vi "(SubVI)Scope_Down Sampling.vi"(7 "Init":bool, 9 "Sampling Time for Init":dbl format="%#_13g", 10 "Iteration":i32, 11 "Data In":i32[][](array[numeric])) -> (1 "end":bool, 2 "Loop Delay (sec)":dbl, 3 "Data Out":i32[][](array[numeric]))   [LabVIEW 2020]
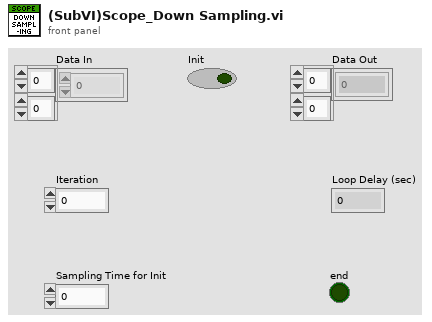
[diagram p1: front panel]
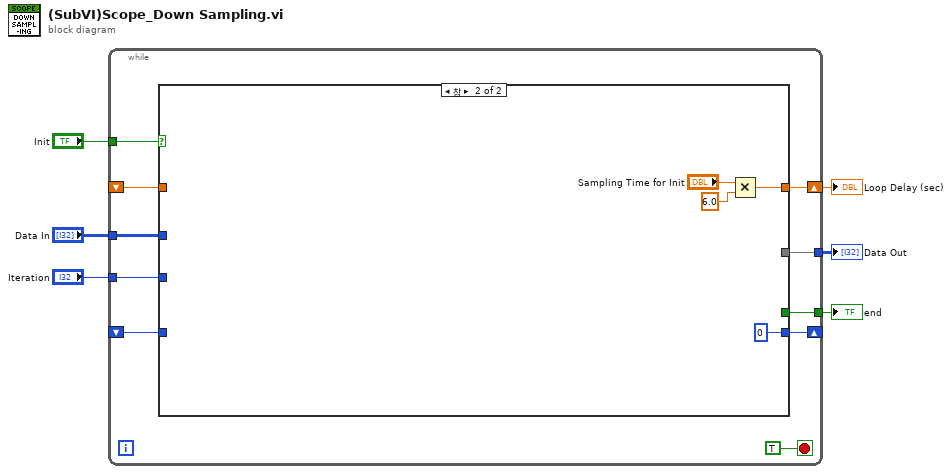
[diagram p0: block diagram]
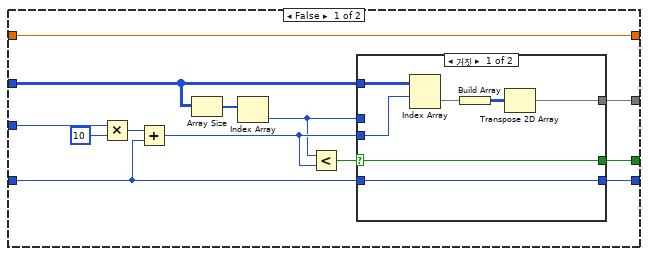
[diagram p2: hidden frame]
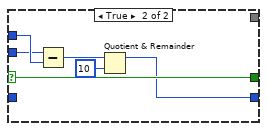
[diagram p3: hidden frame]
diagram:
  n1 = while {
    tunnel: "Init" -> [w15]
    shift-right: [w14] -> w5
    shift-left: _ -> [w13]
    tunnel: "Data In" -> [w12]
    tunnel: "Iteration" -> [w11]
    tunnel: [w10] -> w2
    shift-right: [w8] -> _
    shift-left: _ -> [w9]
    tunnel: [w7] -> w1
    stop <- TRUE stop-if-true
    n2 = case shown="참" w15 {
      tunnel: [w29 w46] -> w14
      tunnel: w13 -> [w29 _]
      tunnel: w12 -> [w24 _]
      tunnel: w11 -> [w28 _]
      tunnel: [w25 _] -> w10
      tunnel: w9 -> [w17 _]
      tunnel: [w18 0] -> w8
      tunnel: [w20 _] -> w7
      frame False {
        n3 = Multiply(x=w28, y=10) -> (x*y=w27:i32)
        n4 = Add(x=w27, y=w17) -> (x+y=w22:i32)
        n5 = Array Size(array=w24) -> (size(s)=w23:i32[])
        n6 = Index Array(array=w23) -> (element=w19:i32)  [unwired: 1 in]
        n7 = Less?(x=w19, y=w22) -> (x < y?=w21:bool)
        n8 = case shown="거짓" w21 {
          selector: w21 -> [w31 w42]
          tunnel: [w34 _] -> w25
          tunnel: w24 -> [w33 _]
          tunnel: w22 -> [w32 w40]
          tunnel: [w31 w42] -> w20
          tunnel: w19 -> [_ w41]
          tunnel: [w30 w38] -> w18
          tunnel: w17 -> [w30 _]
          frame False {
            n9 = Index Array(array=w33, index (row)=w32) -> (element=w36:i32[])  [unwired: 1 in]
            n10 = Build Array(w36) -> (w35:i32[][])
            n11 = Transpose 2D Array(2D array=w35) -> (transposed array=w34:i32[][])
          }
          frame True {
            n12 = Subtract(x=w40, y=w41) -> (x-y=w39:i32)
            n13 = Quotient & Remainder(x=w39, y=10) -> (x-y*floor(x/y)=w38:i32)  [unwired: 1 out]
          }
        }
      }
      frame True {
        n14 = Multiply(x="Sampling Time for Init", y=6.0) -> (x*y=w46:dbl)
      }
    }
  }
  "Loop Delay (sec)" <- w5
  "Data Out" <- w2
  "end" <- w1
